vi "test_CCDIsOpen.vi"() -> ()   [LabVIEW 2023]
uses:
  <vilib>/addons/_JKI Toolkits/Caraya/classes/Test/Test.lvclass
  <vilib>/addons/_JKI Toolkits/Caraya/classes/Assert/Assert.lvclass
  <vilib>/addons/_JKI Toolkits/Caraya/classes/Assert/Assert Equal Value_Variant.vi
  CCD.lvclass
  ccdCount.ctl
panel:
  out "CCD count":T1
  out "error out":errorcluster
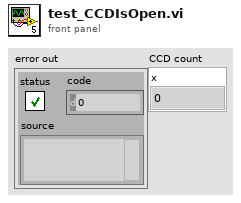
[diagram p1: front panel]
types:
  T1 = typedef "CCD.lvclass/ccdCount.ctl" = cluster{"x":i32}
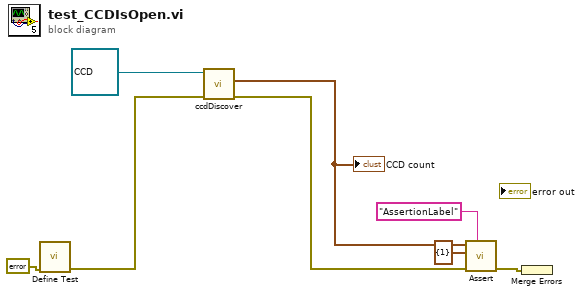
[diagram p0: block diagram]
diagram:
  n1 = call <vilib>:"Define Test.vi"("error in (no error)"=errorcluster {"status"=FALSE, "code"=0, "source"=""}) -> ("error out"=w4:errorcluster)  [unwired: 9 in, 1 out]
  n2 = call "ccdDiscover.vi"("error in (no error)"=w4, "CCD in"=refnum<class "CCD.lvclass"> refnum) -> ("error out"=w3:errorcluster, "CCD count"=w2:T1)  [unwired: 7 in, 1 out]
  "CCD count" <- w2
  n3 = call-poly <vilib>:"Assert.vi"("Label"="AssertionLabel" ("Label (VI Title)"), "error in (no error)"=w3, "Y"=T1 {"x"=1} ("CCD count"), "X"=w2) -> ("error out"=w7:errorcluster)  [unwired: 6 in, 1 out]
  n4 = Merge Errors(w7) -> ()  [unwired: 1 out]
